vi "ShoulderExecuteLogic.vi"(8 "error in (no error)":errorcluster, 10 "LowLimitSwitch":bool, 11 "PositionDeg":dbl) -> (0 "error out":errorcluster, 3 "MotorDemand":dbl)   [LabVIEW 2023]
doc: "Arm Execute for 2024 robot"
uses:
  ShoulderGetSetpointEnum.ctl
  <vilib>/Rock Robotics/WPI/ThirdParty/JAS_Junk/TrajLib/VI/BoolCmd_Recv_Internal.vi
  <vilib>/Rock Robotics/WPI/ThirdParty/JAS_Junk/TrajLib/VI/BoolCmd_ObtainQueue.vi
  ShoulderGlobal.vi
  <vilib>/Rock Robotics/WPI/ThirdParty/JAS_Junk/TrajLib/Trajectory_Library.lvlib
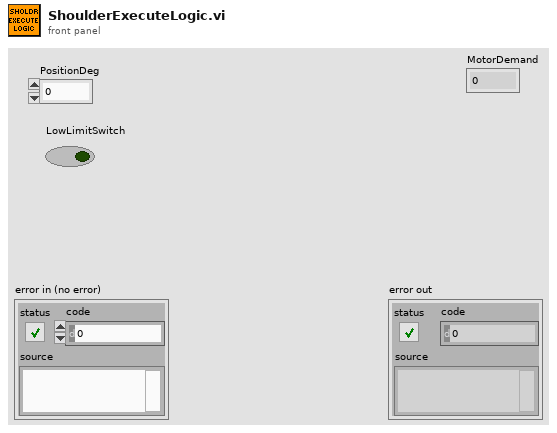
[diagram p1: front panel]
types:
  T1 = typedef "ShoulderGetSetpointEnum.ctl" = enum16{"ShoulderRest", "ShoulderSpeaker", "ShoulderAmp"}
  T2 = typedef "Trajectory_Library.lvlib/PosCtrl_Tuning_Type.ctl" = cluster{"Slope":dbl, "Offset":dbl, "Error Deadband":dbl, "At Reference Count":i32, "Negate Output":bool, "Max Allowd Position":dbl, "Min Allowd Position":dbl}
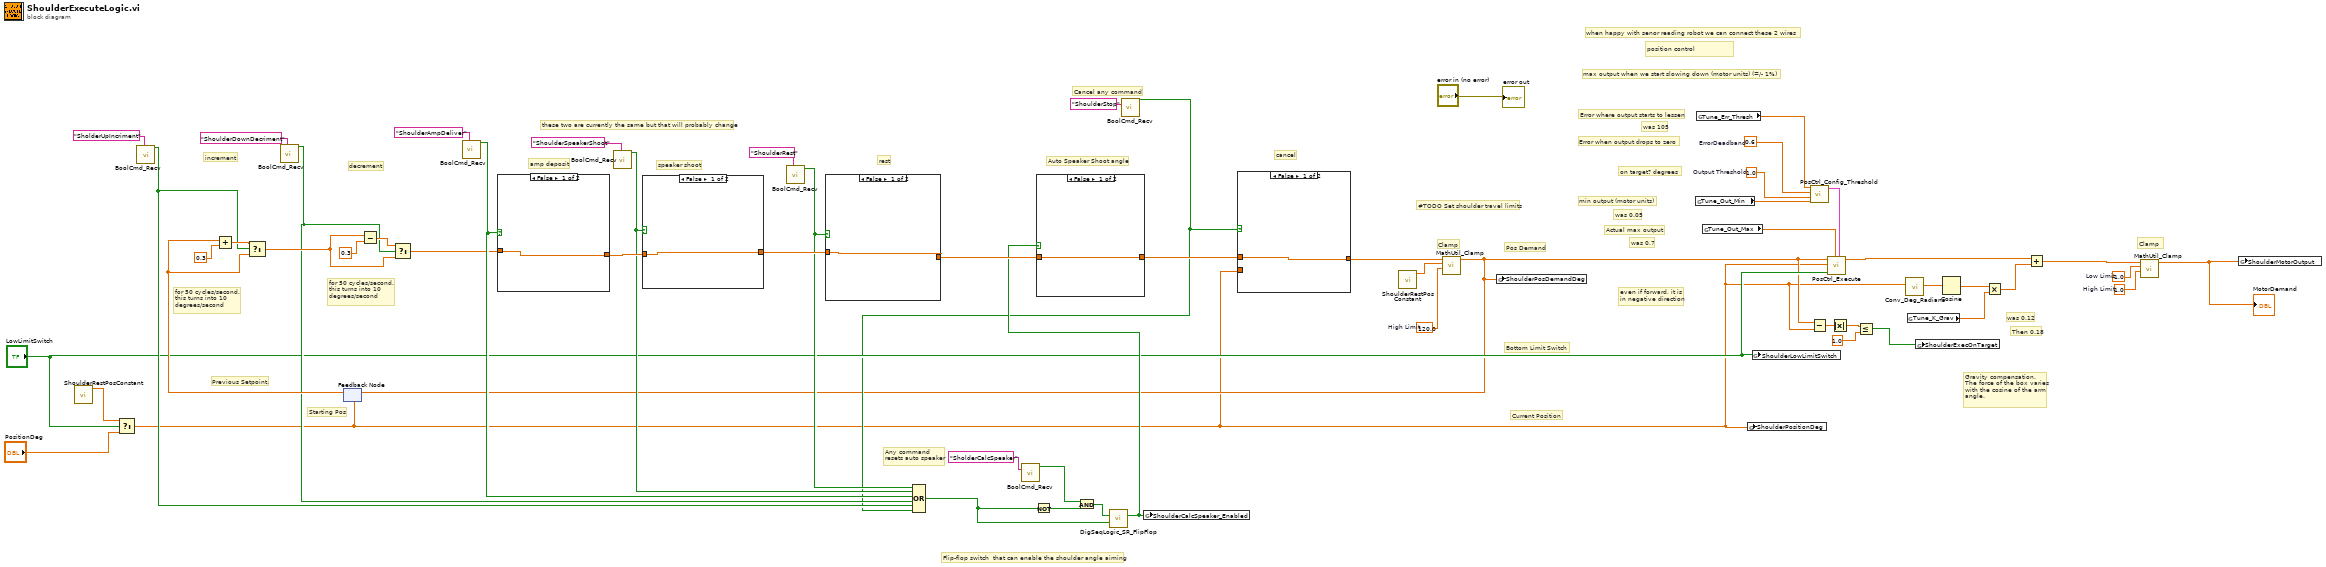
[diagram p0: block diagram]
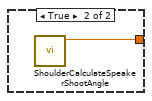
[diagram p2: hidden frame]
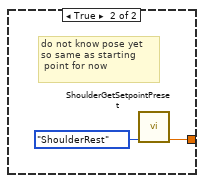
[diagram p4: hidden frame]
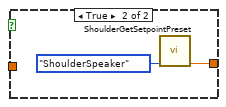
[diagram p5: hidden frame]
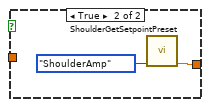
[diagram p6: hidden frame]
diagram:
  w35 = 120.0  # High Limit
  w41 = 1.0  # High Limit
  w40 = -1.0  # Low Limit
  w56 = 0.6  # ErrorDeadband
  w55 = 1.0  # Output Threshold
  # "was 0.05"
  # "was 0.7"
  # "Actual max output"
  # "Then 0.18"
  # "was 0.12"
  # "Previous Setpoint."
  # "Current Position"
  # "Bottom Limit Switch"
  # "Starting Pos"
  # "#TODO Set shoulder travel limits"
  # "Auto Speaker Shoot angle"
  # "Any command\nresets auto speaker"
  # "for 50 cycles/second.\nthis turns into 10 \ndegrees/second"
  # "for 50 cycles/second.\nthis turns into 10 \ndegrees/second"
  # "increment"
  # "Flip-flop switch  that can enable the shoulder angle aiming"
  # "Pos Demand"
  # "Clamp"
  # "was 105"
  # "Gravity compensation.\nThe force of the box varies\nwith the cosine of the arm\nangle."
  # "even if forward, it is \nin negative direction"
  # "these two are currently the same but that will probably change"
  # "Cancel any command"
  # "cancel"
  # "rest"
  # "speaker shoot"
  # "Clamp"
  # "amp deposit"
  # "decrement"
  # "when happy with senor reading robot we can connect these 2 wires"
  # "min output (motor units)"
  # "max output when we start slowing down (motor units) (=/- 1%)"
  # "on target? degrees"
  # "Error when output drops to zero"
  # "position control"
  # "Error where output starts to lessen"
  n1 = call "ShoulderRestPosConstant.vi"() -> ("RestPosition"=w1:dbl)  [unwired: 11 in]
  n2 = Select(t=w1, s="LowLimitSwitch", f="PositionDeg") -> (s? t:f=w11:dbl)
  n3 = call <vilib>:"BoolCmd_Recv.vi"("Command Name"="SholderUpIncriment") -> ("New Request"=w22:bool)  [unwired: 9 in, 1 out]
  n4 = call <vilib>:"BoolCmd_Recv.vi"("Command Name"="ShoulderDownDecriment") -> ("New Request"=w23:bool)  [unwired: 9 in, 1 out]
  n5 = feedback #1(w11) -> (w54:dbl)
  n6 = Add(x=w54, y=0.3) -> (x+y=w32:dbl)
  n7 = Select(t=w32, s=w22, f=w54) -> (s? t:f=w31:dbl)
  n8 = Subtract(x=w31, y=0.3) -> (x-y=w29:dbl)
  n9 = Select(t=w29, s=w23, f=w31) -> (s? t:f=w18:dbl)
  n10 = call <vilib>:"BoolCmd_Recv.vi"("Command Name"="ShoulderAmpDeliver") -> ("New Request"=w24:bool)  [unwired: 9 in, 1 out]
  n11 = case shown="False" w24 {
    tunnel: w18 -> [w58 _]
    tunnel: [w58 w59] -> w53
    frame False {
    }
    frame True {
      n12 = call "ShoulderGetSetpointPreset.vi"("SholdrSetpoints"=ShoulderGetSetpointEnum."ShoulderAmp" ("ArmSetpoints")) -> ("Setpoint"=w59:dbl)  [unwired: 10 in]
    }
  }
  n13 = call <vilib>:"BoolCmd_Recv.vi"("Command Name"="ShoulderSpeakerShoot") -> ("New Request"=w25:bool)  [unwired: 9 in, 1 out]
  n14 = case shown="False" w25 {
    tunnel: w53 -> [w61 _]
    tunnel: [w61 w63] -> w34
    frame False {
    }
    frame True {
      n15 = call "ShoulderGetSetpointPreset.vi"("SholdrSetpoints"=ShoulderGetSetpointEnum."ShoulderSpeaker") -> ("Setpoint"=w63:dbl)  [unwired: 10 in]
    }
  }
  n16 = call <vilib>:"BoolCmd_Recv.vi"("Command Name"="ShoulderRest") -> ("New Request"=w26:bool)  [unwired: 9 in, 1 out]
  n17 = case shown="False" w26 {
    tunnel: w34 -> [w64 _]
    tunnel: [w64 w66] -> w28
    frame False {
    }
    frame True {
      # "do not know pose yet \nso same as starting\n point for now"
      n18 = call "ShoulderGetSetpointPreset.vi"("SholdrSetpoints"=ShoulderGetSetpointEnum."ShoulderRest") -> ("Setpoint"=w66:dbl)  [unwired: 10 in]
    }
  }
  n19 = call <vilib>:"BoolCmd_Recv.vi"("Command Name"="SholderCalcSpeaker") -> ("New Request"=w27:bool)  [unwired: 9 in, 1 out]
  n20 = call <vilib>:"BoolCmd_Recv.vi"("Command Name"="ShoulderStop") -> ("New Request"=w13:bool)  [unwired: 9 in, 1 out]
  n21 = Compound Arithmetic op=OR(w26, w25, w24, w23, w22, w13) -> (w21:bool)
  n22 = Not(x=w21) -> (.not. x?=w37:bool)
  n23 = And(x=w27, y=w37) -> (x .and. y?=w36:bool)
  n24 = call <vilib>:"DigSeqLogic_SR_FlipFlop.vi"("Set"=w36, "Reset"=w21) -> ("Output"=w19:bool)  [unwired: 12 in, 1 out]
  n25 = case shown="False" w19 {
    tunnel: w28 -> [w67 _]
    tunnel: [w67 w68] -> w20
    frame False {
    }
    frame True {
      n26 = call "ShoulderCalculateSpeakerShootAngle.vi"() -> ("ShoulderDesiredAngle (degrees)"=w68:dbl)  [unwired: 11 in]
    }
  }
  n27 = global write "ShoulderGlobal.vi" "ShoulderCalcSpeaker_Enabled"(w19) -> ()
  n28 = case shown="False" w13 {
    tunnel: w20 -> [w69 _]
    tunnel: [w69 w70] -> w16
    tunnel: w11 -> [_ w70]
    frame False {
    }
    frame True {
      # "takes get sensor pose pose"
    }
  }
  n29 = call "ShoulderRestPosConstant.vi"() -> ("RestPosition"=w2:dbl)  [unwired: 11 in]
  n30 = call <vilib>:"MathUtil_Clamp.vi"("High Limit"=w35, "Low Limit"=w2, "Value"=w16) -> ("Result"=w12:dbl)  [unwired: 8 in]
  n31 = feedback-in #1(w12) -> ()
  n32 = global write "ShoulderGlobal.vi" "ShoulderPosDemandDeg"(w12) -> ()
  n33 = global read "ShoulderGlobal.vi" "Tune_Out_Min"() -> (w4:dbl)
  n34 = global read "ShoulderGlobal.vi" "Tune_Err_Thresh"() -> (w3:dbl)
  n35 = global read "ShoulderGlobal.vi" "Tune_Out_Max"() -> (w5:dbl)
  n36 = global write "ShoulderGlobal.vi" "ShoulderPositionDeg"(w11) -> ()
  n37 = global write "ShoulderGlobal.vi" "ShoulderLowLimitSwitch"("LowLimitSwitch") -> ()
  n38 = call <vilib>:"PosCtrl_Config_Threshold.vi"("Output Deadband"=w4, "Output Threshold"=w55, "ErrorDeadband"=w56, "ErrorThreshold"=w3) -> ("PosCtrl_Config_Params"=w57:T2)  [unwired: 7 in]
  n39 = Subtract(x=w12, y=w11) -> (x-y=w10:dbl)
  n40 = call <vilib>:"PosCtrl_Execute.vi"("PosCtrl_Config_Params"=w57, "MaxOutput"=w5, "Rev Limit Switch"="LowLimitSwitch", "CurrentPosition"=w11, "TargetPosition"=w12) -> ("Output"=w45:dbl)  [unwired: 4 in, 2 out]
  n41 = Absolute Value(x=w10) -> (abs(x)=w9:dbl)
  n42 = Less Or Equal?(x=w9, y=1.0) -> (x <= y?=w7:bool)
  n43 = call <vilib>:"Conv_Deg_Radians.vi"("Degress"=w11) -> ("Radians"=w42:dbl)  [unwired: 10 in]
  n44 = global read "ShoulderGlobal.vi" "Tune_K_Grav"() -> (w6:dbl)
  n45 = global write "ShoulderGlobal.vi" "ShoulderExecOnTarget"(w7) -> ()
  n46 = Cosine(x=w42) -> (cos(x)=w43:dbl)
  n47 = Multiply(x=w43, y=w6) -> (x*y=w44:dbl)
  n48 = Add(x=w45, y=w44) -> (x+y=w39:dbl)
  n49 = call <vilib>:"MathUtil_Clamp.vi"("High Limit"=w41, "Low Limit"=w40, "Value"=w39) -> ("Result"=w14:dbl)  [unwired: 8 in]
  "MotorDemand" <- w14
  n50 = global write "ShoulderGlobal.vi" "ShoulderMotorOutput"(w14) -> ()
  "error out" <- "error in (no error)"
